vi "Kpro Read String Pot 2016.vi"(0 "Read String Pot":bool, 1 "Feet of\nStainless to be\nUsed (Count) in":i32, 2 "Session Array in":dbl[][](array[numeric]), 3 "Flow":dbl, 4 "Manual Depth In":dbl, 5 "Finished In":bool, 6 "Depth Cluster in":T1, 7 "error in (no error)":errorcluster, 8 "String Pot \nSlope in":dbl=1.7339999675750732 format="%.2f", 9 "Sensor Cluster In in":T2, 10 "Descriptions":string[](array[string]), 11 "Pressure in":dbl format="%.2f", 12 "Array in":refnum<k24>[](array[refnum]), 13 "Downhole Pressure Sensor":dbl format="%#_13g") -> (18 "Sensor Cluster 2":T2, 19 "IK":dbl, 20 "Array out":refnum<k24>[](array[refnum]), 21 "Generate Array Calc IK":bool, 22 "Finish Take Data":bool, 23 "Depth Rate":dbl format="%.2f", 24 "Feet of\nStainless to be\nUsed (Count) out":i32, 25 "Depth Cluster out":T1, 26 "Single String Pot Session Array out":dbl[][](array[numeric]))   [LabVIEW 2016]
uses:
  controls/MCC DAQ Readings.ctl
  C:/Program Files (x86)/National Instruments/LabVIEW 2016/vi.lib/ULx/ULx_LV.dll
  controls/Kpro hydraulic measurement cluster.ctl
panel:
  out "Manual measurement triggered":bool
  out "Filter Output":dbl
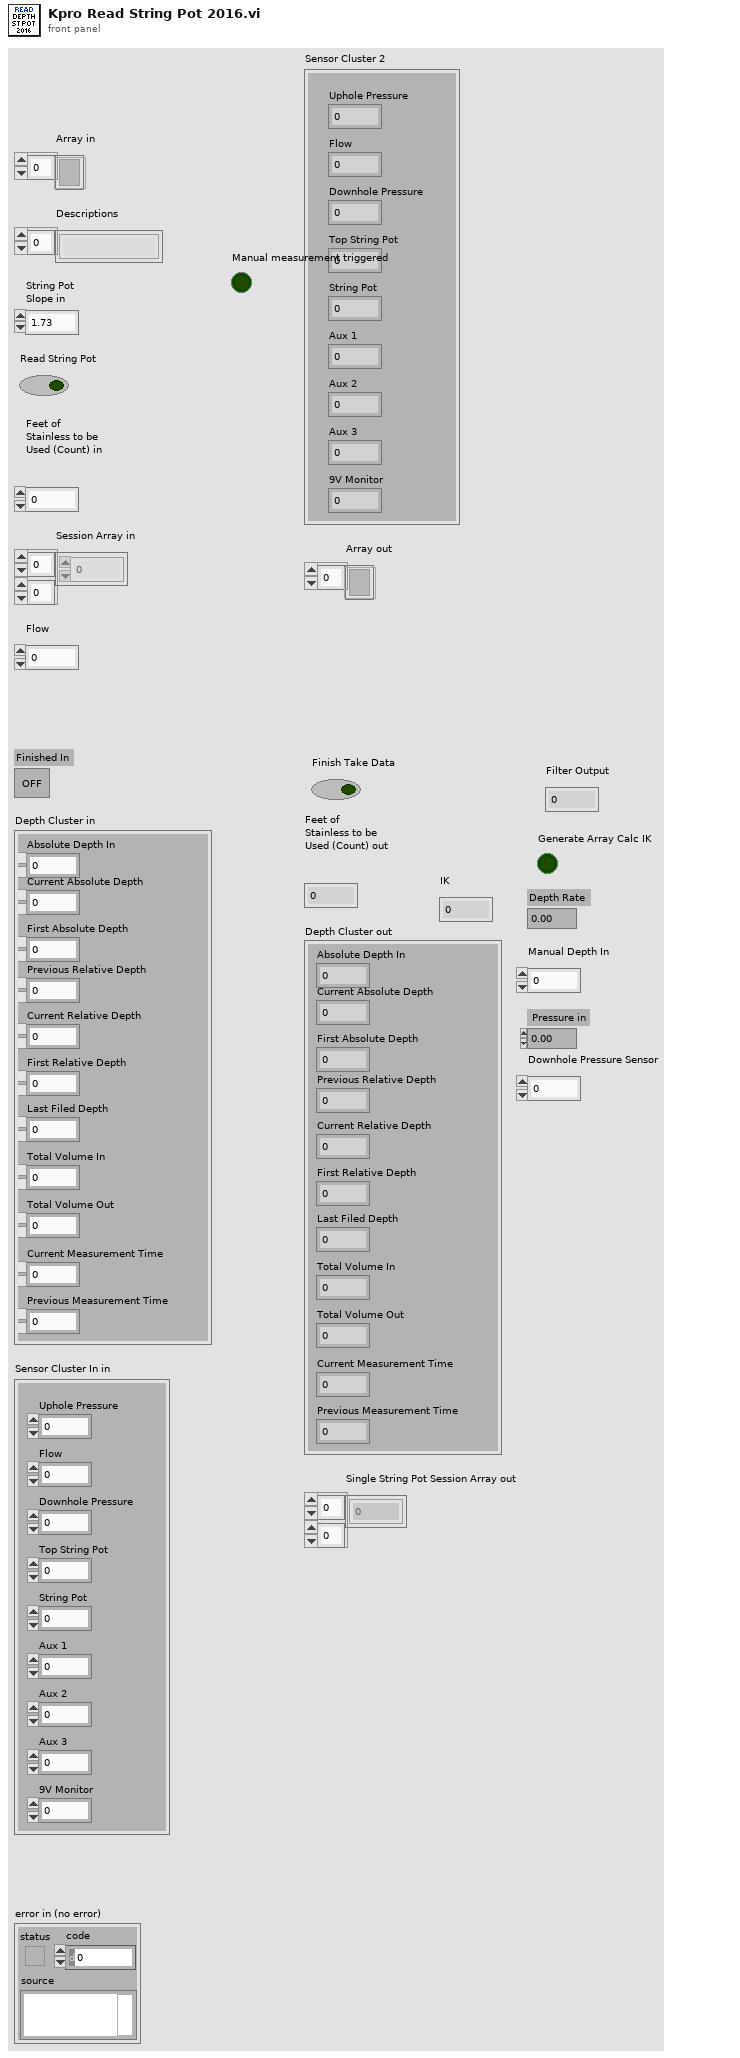
[diagram p1: front panel]
types:
  T1 = typedef "Kpro hydraulic measurement cluster.ctl" = cluster{"Absolute Depth In":dbl, "Current Absolute Depth":dbl, "First Absolute Depth":dbl, "Previous Relative Depth":dbl, "Current Relative Depth":dbl, "First Relative Depth":dbl, "Last Filed Depth":dbl, "Total Volume In":dbl, "Total Volume Out":dbl, "Current Measurement Time":dbl, "Previous Measurement Time":dbl}
  T2 = typedef "MCC DAQ Readings.ctl" = cluster{"Uphole Pressure":dbl, "Flow":dbl, "Downhole Pressure":dbl, "Top String Pot":dbl, "String Pot":dbl, "Aux 1":dbl, "Aux 2":dbl, "Aux 3":dbl, "9V Monitor":dbl}
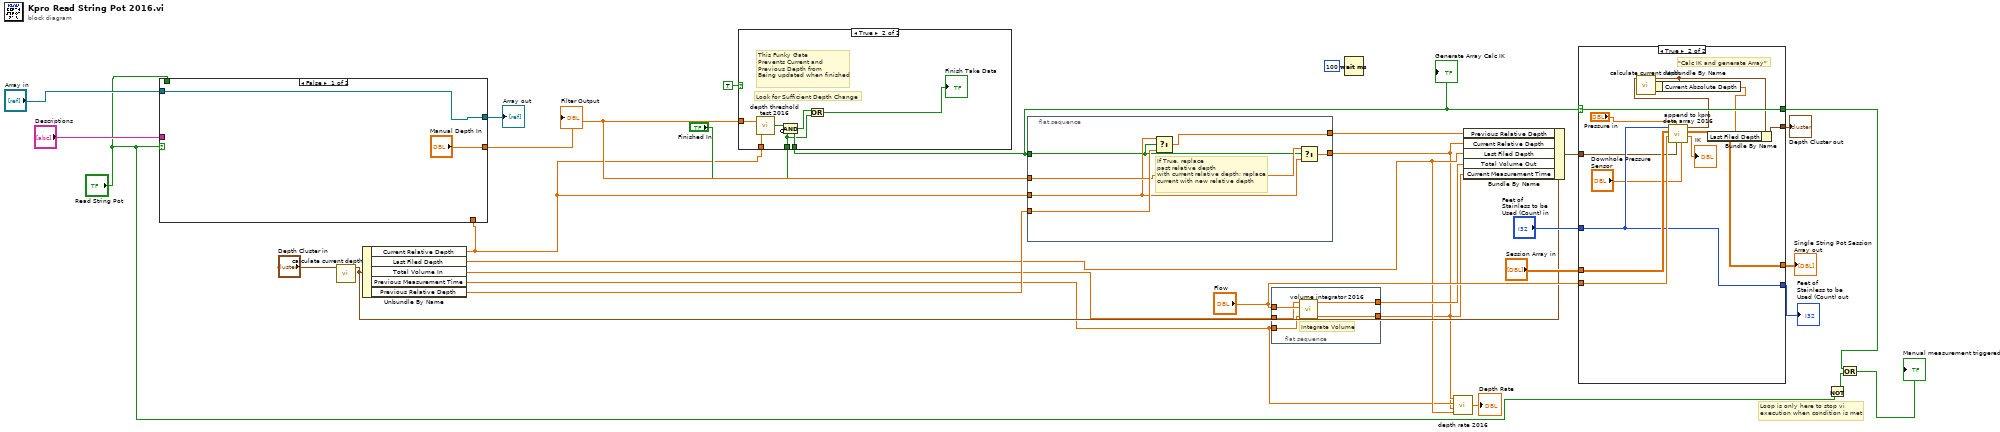
[diagram p0: block diagram]
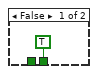
[diagram p2: hidden frame]
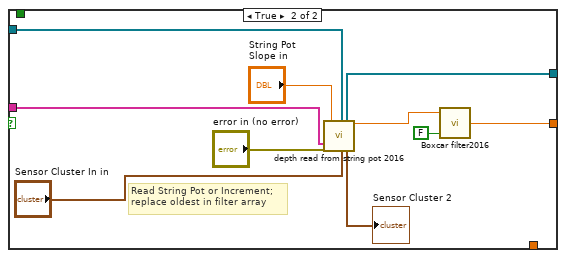
[diagram p3: hidden frame]
diagram:
  # "Loop is only here to stop vi \nexecution when condition is met"
  n1 = call "calculate current depth.vi"("Cluster in"="Depth Cluster in") -> ("Cluster out"=w21:T1)  [unwired: 10 in]
  n2 = Unbundle By Name(w21) -> ("Current Relative Depth"=w8:dbl, "Last Filed Depth"=w11:dbl, "Total Volume In"=w16:dbl, "Previous Measurement Time"=w9:dbl, "Previous Relative Depth"=w19:dbl)
  n3 = case shown="False" "Read String Pot" {
    tunnel: ["Manual Depth In" w42] -> w15
    tunnel: "Read String Pot" -> [_ _]
    tunnel: "Descriptions" -> [_ w41]
    tunnel: [w33 w38] -> w30
    tunnel: "Array in" -> [w33 w37]
    tunnel: w8 -> [_ _]
    frame False {
    }
    frame True {
      # "Read String Pot or Increment;\nreplace oldest in filter array"
      n4 = call "depth read from string pot 2016.vi"("Descriptions"=w41, "error in (no error)"="error in (no error)", "String Pot \nSlope"="String Pot \nSlope in", "Array in"=w37, "Sensor Cluster In"="Sensor Cluster In in") -> ("Array out"=w38:refnum<k24>[], "Sensor Cluster 2"=→"Sensor Cluster 2":T2, "Depth"=w43:dbl)  [unwired: 11 in, 1 out]
      n5 = call "Boxcar filter2016.vi"("Initialize"=FALSE, "Filter Input"=w43) -> ("Filter Output"=w42:dbl)  [unwired: 1 in]
    }
  }
  "Array out" <- w30
  "Filter Output" <- w15
  n6 = case shown="True" TRUE {
    tunnel: [TRUE w49] -> w13
    tunnel: "Finished In" -> [_ w48]
    tunnel: w15 -> [_ w47]
    tunnel: w8 -> [_ w46]
    frame False {
    }
    frame True {
      # "Look for Sufficient Depth Change"
      # "This Funky Gate\nPrevents Current and \nPrevious Depth from \nBeing updated when finished"
      n7 = call "depth threshold test 2016.vi"("Depth\nPrevious"=w46, "Depth \nCurrent"=w47) -> ("Threshold\nExceeded"=w50:bool)
      n8 = Compound Arithmetic op=AND(w50, invert w48) -> (w49:bool)
      n9 = Or(x=w49, y=w48) -> (x .or. y?=→"Finish Take Data":bool)
    }
  }
  "Generate Array Calc IK" <- w13
  n10 = flat-sequence {
    tunnel: [w56] -> w18
    tunnel: w19 -> [w55]
    tunnel: [w54] -> w3
    tunnel: w13 -> [w51]
    tunnel: w15 -> [w53]
    tunnel: w8 -> [w52]
    frame #0 {
      # "If True, replace\npast relative depth\nwith current relative depth; replace\ncurrent with new relative depth"
      n11 = Select(t=w52, s=w51, f=w55) -> (s? t:f=w56:dbl)
      n12 = Select(t=w53, s=w51, f=w52) -> (s? t:f=w54:dbl)
    }
  }
  n13 = flat-sequence {
    tunnel: w9 -> [w61]
    tunnel: [w60] -> w10
    tunnel: "Flow" -> [w59]
    tunnel: w16 -> [w58]
    tunnel: [w57] -> w17
    frame #0 {
      # "Integrate Volume"
      n14 = call "volume integrator 2016.vi"("Previous Time (sec)"=w61, "Flow"=w59, "Total Volume in"=w58) -> ("Current Time (sec)"=w60:dbl, "Total Volume Out mL"=w57:dbl)  [unwired: 3 in]
    }
  }
  n15 = Wait (ms)(milliseconds to wait=u32 100) -> ()  [unwired: 1 out]
  n16 = call "depth rate 2016.vi"("Depth Last"=w11, "Depth Current"=w3, "Time Last"=w9, "Time Current"=w10) -> ("Depth Rate"=→"Depth Rate":dbl)
  n17 = Bundle By Name(cluster=w21, "Previous Relative Depth"=w18, "Current Relative Depth"=w3, "Last Filed Depth"=w11, "Total Volume Out"=w17, "Current Measurement Time"=w10) -> (w22:T1)
  n18 = case shown="True" w13 {
    selector: w13 -> [w63 w71]
    tunnel: "Session Array in" -> [w62 w78]
    tunnel: [w62 w77] -> w25
    tunnel: "Feet of\nStainless to be\nUsed (Count) in" -> [w64 w74]
    tunnel: "Flow" -> [_ w76]
    tunnel: [w65 w70] -> w23
    tunnel: w22 -> [w65 w69]
    tunnel: [w64 w74] -> w28
    tunnel: [w63 w71] -> w7
    frame False {
    }
    frame True {
      # "\"Calc IK and generate Array\""
      n19 = call "append to kpro data array 2016.vi"("Downhole Pressure Sensor"="Downhole Pressure Sensor", "Cluster in"=w69, "Up hole Pressure Sensor"="Pressure in", "Flow"=w76, "Corrected Array in"=w78, "Feet of\nStainless to be\nUsed (Count) in"=w74) -> ("IK"=→"IK":dbl, "Array Out"=w77:dbl[][], "Cluster out 2"=w68:T1)  [unwired: 2 in, 1 out]
      n20 = call "calculate current depth.vi"("Cluster in"=w68) -> ("Cluster out"=w67:T1)  [unwired: 10 in]
      n21 = Unbundle By Name(w67) -> ("Current Absolute Depth"=w66:dbl)
      n22 = Bundle By Name(cluster=w67, "Last Filed Depth"=w66) -> (w70:T1)
    }
  }
  "Feet of\nStainless to be\nUsed (Count) out" <- w28
  "Single String Pot Session Array out" <- w25
  "Depth Cluster out" <- w23
  n23 = Not(x="Read String Pot") -> (.not. x?=w4:bool)
  n24 = Or(x=w7, y=w4) -> (x .or. y?=→"Manual measurement triggered":bool)
